vi "UHR-Fleezers Control (host) - 10.6.vi"() -> ()   [LabVIEW 2011] (continued)
        n1265 = Open/Create/Replace File(file path (use dialog)=w1906, operation (0:open)=T25."open", access (0:read/write)=enum16{"read/write", "read-only", "write-only"}."read-only") -> (refnum out=w1914:refnum<file>, error out=w1900:errorcluster)  [unwired: 1 in, 3 out]
        n1266 = Deny Access(4:w1900, 7:w1914) -> (0:w1899:errorcluster, 3:w1905:refnum<file>)  [unwired: 1 out]
        n1267 = Read from Binary File(5:0.0, 8:w1899, 9:T24."big-endian, network order" ("byte order (0:big-endian, network order)"), 10:-1 ("count (1)"), 11:w1905) -> (0:w1898:errorcluster, 2:w1896:dbl[], 3:w1901:refnum<file>)  [unwired: 2 out]
        n1268 = Array To Cluster(array=w1896) -> (cluster=w1895:T27)
        n1269 = Unbundle(w1895) -> ("[0]"=w1894:dbl, "[1]"=w1893:dbl, "[2]"=w1892:dbl, "[3]"=w1891:dbl, "[4]"=w1890:dbl, "[5]"=w1889:dbl)
        n1270 = Close File(refnum=w1901, error in=w1898) -> (error out=→"Read cal error":errorcluster)  [unwired: 1 out]
        n1271 = Multiply(x=w1889, y=w1886) -> (x*y=w1887:dbl)
        n1272 = local write "T2 kappa_x (pN/nm)"(w1891) -> ()
        n1273 = local write "T1 kappa_x (pN/nm)"(w1892) -> ()
        n1274 = local write "T1 alpha_x (nm/V)"(w1894) -> ()
        n1275 = local write "T2 alpha_x (nm/V)"(w1893) -> ()
        n1276 = Multiply(x=w1890, y=w1886) -> (x*y=w1888:dbl)
        n1277 = local write "T1 offset_x (mV)"(w1888) -> ()
        n1278 = local write "T2 offset_x (mV)"(w1887) -> ()
      }
      event "Abort MCL Scan": Value Change {
        n1279 = event-data() -> ()  [unwired: 7 out]
        n1280 = local write "MCL Scanning"(FALSE ("MCL Scanning")) -> ()
        n1281 = xnode "Read/Write Control"("FPGA VI Reference In"=w1919, "error in"=w1918, "Abort scan (MCL)"="Abort MCL Scan") -> ("error out"=w1917:errorcluster)  [unwired: 1 out]
      }
      event "Update Count (MCL)": Value Change {
        n1282 = event-data() -> ()  [unwired: 7 out]
        n1283 = xnode "Read/Write Control"("FPGA VI Reference In"=w1923, "error in"=w1922, "MCL count"="Update Count (MCL)") -> ("error out"=w1921:errorcluster)  [unwired: 1 out]
      }
      event "Phase adjust (MCL)", "+ phase (MCL)", "- phase (MCL)": Value Change {
        n1284 = event-data() -> ()  [unwired: 7 out]
        n1285 = Negate(x="Phase adjust (MCL)") -> (-x=w1932:i16)
        n1286 = Select(t=w1932, s="- phase (MCL)", f="Phase adjust (MCL)") -> (s? t:f=w1930:i16)
        n1287 = Or(x="- phase (MCL)", y="+ phase (MCL)") -> (x .or. y?=w1925:bool)
        n1288 = xnode "Read/Write Control"("FPGA VI Reference In"=w1934, "error in"=w1933, "Phase count adjustment (MCL)"=w1930) -> ("FPGA VI Reference Out"=w1926:T19, "error out"=w1927:errorcluster)
        n1289 = xnode "Read/Write Control"("FPGA VI Reference In"=w1926, "error in"=w1927, "+ phase (MCL)"=w1925) -> ("error out"=w1924:errorcluster)  [unwired: 1 out]
      }
      event "Abort AOD Scan": Value Change {
        n1290 = event-data() -> ()  [unwired: 7 out]
        n1291 = xnode "Read/Write Control"("FPGA VI Reference In"=w1938, "error in"=w1937, "Abort scan"="Abort AOD Scan") -> ("error out"=w1936:errorcluster)  [unwired: 1 out]
      }
      event "Continuous AOD Scanning": Value Change {
        n1292 = event-data() -> ()  [unwired: 7 out]
        n1293 = xnode "Read/Write Control"("FPGA VI Reference In"=w1942, "error in"=w1941, "Cont. Scan"="Continuous AOD Scanning") -> ("error out"=w1940:errorcluster)  [unwired: 1 out]
      }
      event "Index": Value Change {
        n1294 = event-data() -> ()  [unwired: 7 out]
        n1295 = call "Create new save file.vi"("Insert"="", "Ext"=".dat" ("string"), "Index In"="Index") -> ("Path Out"=→"Save file name":path, "Index Out"=w1943:dbl)
        "Save index" <- w1943
        n1296 = local write "Index"(w1943) -> ()
      }
      event "AO1", "AO2": Value Change {
        w1958 = 10.0 ("y")
        w1957 = 32767.0 ("y")
        n1297 = event-data() -> ()  [unwired: 7 out]
        n1298 = local read "AO2"() -> (w1956:dbl)
        n1299 = local read "AO1"() -> (w1953:dbl)
        n1300 = Multiply(x=w1953, y=w1957) -> (x*y=w1952:dbl)
        n1301 = Multiply(x=w1956, y=w1957) -> (x*y=w1955:dbl)
        n1302 = Divide(x=w1952, y=w1958) -> (x/y=w1951:dbl)
        n1303 = Divide(x=w1955, y=w1958) -> (x/y=w1954:dbl)
        n1304 = To Word Integer(number=w1951) -> (16bit integer=w1959:i16)
        n1305 = To Word Integer(number=w1954) -> (16bit integer=w1960:i16)
        n1306 = xnode "Read/Write Control"("FPGA VI Reference In"=w1950, "error in"=w1949, "AO1"=w1959, "AO2"=w1960) -> ("error out"=w1948:errorcluster)  [unwired: 1 out]
      }
      event "Inject Pump 1": Value Change {
        n1307 = event-data() -> ()  [unwired: 7 out]
        n1308 = local read "Use Harvard pumps\nfor beads (else Chemyx)"() -> (w1962:bool)
        n1309 = case shown="True" w1962 {
          tunnel: "Inject Pump 1" -> [w1966 w2004]
          tunnel: w1961 -> [_ w2005]
          frame False {
            n1310 = local read "Pump write delay (ms)"() -> (w1965:dbl)
            n1311 = local read "Chemyx Syringe Pump Serial Port"() -> (w1964:refnum<visa-resource-name>)
            n1312 = case shown="True" w1966 {
              tunnel: w1965 -> [w1972 w1986]
              tunnel: w1964 -> [w1969 w1985]
              frame False {
                n1313 = flat-sequence {
                  tunnel: w1969 -> [w1973]
                  tunnel: [w1973] -> w1970
                  tunnel: w1972 -> [_]
                  tunnel: [w1976] -> w1971
                  tunnel: w1970 -> [w1976]
                  tunnel: w1971 -> [w1977]
                  tunnel: [w1977] -> w1967
                  tunnel: [w1979] -> w1968
                  tunnel: w1967 -> [w1979]
                  tunnel: w1968 -> [w1981]
                  frame #0 {
                    n1314 = call "Write to pump.vi"("string"="enter pump1", "VISA resource name"=w1973) -> ()  [unwired: 1 out]
                  }
                  frame #1 {
                    n1315 = Wait (ms)(milliseconds to wait="Pump pause delay (ms)") -> ()  [unwired: 1 out]
                  }
                  frame #2 {
                    n1316 = call "Write to pump.vi"("string"="stop", "VISA resource name"=w1977) -> ()  [unwired: 1 out]
                  }
                  frame #3 {
                    n1317 = Wait (ms)(milliseconds to wait=u32 500) -> ()  [unwired: 1 out]
                  }
                  frame #4 {
                    n1318 = call "Write to pump.vi"("string"="stop", "VISA resource name"=w1981) -> ()  [unwired: 1 out]
                  }
                }
              }
              frame True {
                n1319 = flat-sequence {
                  tunnel: w1985 -> [w1995]
                  tunnel: w1986 -> [w1990]
                  tunnel: w1986 -> [w1997]
                  tunnel: w1985 -> [w1998]
                  tunnel: [w1998] -> w1983
                  tunnel: [w2000] -> w1984
                  tunnel: w1983 -> [w2000]
                  tunnel: w1984 -> [w2002]
                  frame #0 {
                    n1320 = local read "All Pump Parameters"() -> (w1989:T5)
                    n1321 = Unbundle By Name(w1989) -> ("Pump 1"=w1996:T28)
                    n1322 = call "Set pump parameters.vi"("Pump write delay (ms)"=w1990, "Volume (uL)"="Ch 1 Inject Volume (uL)", "Rate (uL/h)"="Ch 1 Inject Rate (ul/h)", "Units"=4.0, "Pump #"=1.0, "Pump Parameters In"=w1996, "VISA resource name"=w1995) -> ("Pump Parameters Out"=w1988:T28)  [unwired: 3 in]
                    n1323 = Bundle By Name(cluster=w1989, "Pump 1"=w1988) -> (w1987:T5)
                    n1324 = local write "All Pump Parameters"(w1987) -> ()
                  }
                  frame #1 {
                    n1325 = Wait (ms)(milliseconds to wait=w1997) -> ()  [unwired: 1 out]
                  }
                  frame #2 {
                    n1326 = call "Write to pump.vi"("string"="start", "VISA resource name"=w1998) -> ()  [unwired: 1 out]
                  }
                  frame #3 {
                    n1327 = Wait (ms)(milliseconds to wait=u32 500) -> ()  [unwired: 1 out]
                  }
                  frame #4 {
                    n1328 = call "Write to pump.vi"("string"="start", "VISA resource name"=w2002) -> ()  [unwired: 1 out]
                  }
                }
              }
            }
          }
          frame True {
            n1329 = case shown="False" w2004 {
              tunnel: w2005 -> [w2006 w2016]
              frame False {
                n1330 = flat-sequence {
                  tunnel: w2006 -> [w2008]
                  frame #0 {
                    n1331 = local write "Flushing P1"(FALSE ("Flushing P1")) -> ()
                    n1332 = Concatenate Strings("stop" ("string"), "\r") -> (w2010:string)
                    n1333 = VISA Write(VISA resource name=w2008, write buffer=w2010) -> ()  [unwired: 1 in, 3 out]
                  }
                  frame #1 {
                    n1334 = property on="Clear Volume P1" class="Bool (strict)"("Val(Sgnl)"=TRUE ("Value (Signaling)")) -> ()  [unwired: 2 in, 2 out]
                  }
                }
              }
              frame True {
                n1335 = local read "Normal Flow Rate (ul/h) P1"() -> (w2014:dbl)
                n1336 = Number To Decimal String(number=w2014) -> (decimal integer string=w2020:string)  [unwired: 1 in]
                n1337 = Concatenate Strings("irate  " ("string"), w2020, " u/h" ("string"), "\r") -> (w2018:string)
                n1338 = VISA Write(VISA resource name=w2016, write buffer=w2018) -> (VISA resource name out=w2015:refnum<visa-resource-name>)  [unwired: 1 in, 2 out]
                n1339 = Concatenate Strings("irun" ("string"), "\r") -> (w2022:string)
                n1340 = VISA Write(VISA resource name=w2015, write buffer=w2022) -> ()  [unwired: 1 in, 3 out]
              }
            }
          }
        }
      }
      event "Inject Pump 3": Value Change {
        n1341 = event-data() -> ()  [unwired: 7 out]
        n1342 = local read "Use Harvard pumps\nfor beads (else Chemyx)"() -> (w2025:bool)
        n1343 = case shown="True" w2025 {
          tunnel: "Inject Pump 3" -> [w2029 w2068]
          tunnel: w2024 -> [_ w2067]
          frame False {
            n1344 = local read "Pump write delay (ms)"() -> (w2028:dbl)
            n1345 = case shown="True" w2029 {
              tunnel: w2028 -> [w2035 w2049]
              tunnel: "Chemyx Syringe Pump Serial Port" -> [w2032 w2048]
              frame False {
                n1346 = flat-sequence {
                  tunnel: w2032 -> [w2036]
                  tunnel: [w2036] -> w2033
                  tunnel: w2035 -> [_]
                  tunnel: [w2039] -> w2034
                  tunnel: w2033 -> [w2039]
                  tunnel: w2034 -> [w2040]
                  tunnel: [w2040] -> w2030
                  tunnel: [w2042] -> w2031
                  tunnel: w2030 -> [w2042]
                  tunnel: w2031 -> [w2044]
                  frame #0 {
                    n1347 = call "Write to pump.vi"("string"="enter pump3", "VISA resource name"=w2036) -> ()  [unwired: 1 out]
                  }
                  frame #1 {
                    n1348 = local read "Pump pause delay (ms)"() -> (w2038:u32)
                    n1349 = Wait (ms)(milliseconds to wait=w2038) -> ()  [unwired: 1 out]
                  }
                  frame #2 {
                    n1350 = call "Write to pump.vi"("string"="stop", "VISA resource name"=w2040) -> ()  [unwired: 1 out]
                  }
                  frame #3 {
                    n1351 = Wait (ms)(milliseconds to wait=u32 0) -> ()  [unwired: 1 out]
                  }
                  frame #4 {
                    n1352 = call "Write to pump.vi"("string"="stop", "VISA resource name"=w2044) -> ()  [unwired: 1 out]
                  }
                }
              }
              frame True {
                n1353 = flat-sequence {
                  tunnel: w2048 -> [w2058]
                  tunnel: w2049 -> [w2053]
                  tunnel: w2049 -> [w2060]
                  tunnel: w2048 -> [w2061]
                  tunnel: [w2061] -> w2047
                  tunnel: [w2064] -> w2046
                  tunnel: w2047 -> [w2064]
                  tunnel: w2046 -> [w2065]
                  frame #0 {
                    n1354 = local read "All Pump Parameters"() -> (w2052:T5)
                    n1355 = Unbundle By Name(w2052) -> ("Pump 3"=w2059:T28)
                    n1356 = call "Set pump parameters.vi"("Pump write delay (ms)"=w2053, "Volume (uL)"="Ch 3 Inject Volume (uL)", "Rate (uL/h)"="Ch 3 Inject Rate (ul/h)", "Units"=4.0, "Pump #"=3.0, "Pump Parameters In"=w2059, "VISA resource name"=w2058) -> ("Pump Parameters Out"=w2051:T28)  [unwired: 3 in]
                    n1357 = Bundle By Name(cluster=w2052, "Pump 3"=w2051) -> (w2050:T5)
                    n1358 = local write "All Pump Parameters"(w2050) -> ()
                  }
                  frame #1 {
                    n1359 = Wait (ms)(milliseconds to wait=w2060) -> ()  [unwired: 1 out]
                  }
                  frame #2 {
                    n1360 = call "Write to pump.vi"("string"="start", "VISA resource name"=w2061) -> ()  [unwired: 1 out]
                  }
                  frame #3 {
                    n1361 = Wait (ms)(milliseconds to wait=u32 500) -> ()  [unwired: 1 out]
                  }
                  frame #4 {
                    n1362 = call "Write to pump.vi"("string"="start", "VISA resource name"=w2065) -> ()  [unwired: 1 out]
                  }
                }
              }
            }
          }
          frame True {
            n1363 = case shown="False" w2068 {
              tunnel: w2067 -> [w2069 w2076]
              frame False {
                n1364 = flat-sequence {
                  tunnel: w2069 -> [w2071]
                  frame #0 {
                    n1365 = local write "Flushing P3"(FALSE ("Flushing P3")) -> ()
                    n1366 = Concatenate Strings("stop" ("string"), "\r") -> (w2073:string)
                    n1367 = VISA Write(VISA resource name=w2071, write buffer=w2073) -> ()  [unwired: 1 in, 3 out]
                  }
                  frame #1 {
                    n1368 = property on="Clear Volume P3" class="Bool (strict)"("Val(Sgnl)"=TRUE ("Value (Signaling)")) -> ()  [unwired: 2 in, 2 out]
                  }
                }
              }
              frame True {
                n1369 = local read "Normal Flow Rate (ul/h) P3"() -> (w2077:dbl)
                n1370 = Number To Decimal String(number=w2077) -> (decimal integer string=w2083:string)  [unwired: 1 in]
                n1371 = Concatenate Strings("irate  " ("string"), w2083, " u/h" ("string"), "\r") -> (w2081:string)
                n1372 = VISA Write(VISA resource name=w2076, write buffer=w2081) -> (VISA resource name out=w2079:refnum<visa-resource-name>)  [unwired: 1 in, 2 out]
                n1373 = Concatenate Strings("irun" ("string"), "\r") -> (w2085:string)
                n1374 = VISA Write(VISA resource name=w2079, write buffer=w2085) -> ()  [unwired: 1 in, 3 out]
              }
            }
          }
        }
      }
      event "Inject Pump 2": Value Change {
        n1375 = event-data() -> ()  [unwired: 7 out]
        n1376 = local read "Pump write delay (ms)"() -> (w2089:dbl)
        n1377 = flat-sequence {
          tunnel: w2087 -> [w2102]
          tunnel: w2089 -> [w2098]
          tunnel: "Inject Pump 2" -> [_]
          tunnel: w2089 -> [w2104]
          tunnel: w2087 -> [w2105]
          frame #0 {
            n1378 = local read "All Pump Parameters"() -> (w2097:T5)
            n1379 = Multiply(x=60.0, y="Flush Center Ch Rate (ul/m)") -> (x*y=w2094:dbl)
            n1380 = Unbundle By Name(w2097) -> ("Pump 2"=w2103:T28)
            n1381 = call "Set pump parameters.vi"("Pump write delay (ms)"=w2098, "Volume (uL)"="Flush Center Ch Volume (uL)", "Rate (uL/h)"=w2094, "Units"=3.0, "Pump #"=2.0, "Pump Parameters In"=w2103, "VISA resource name"=w2102) -> ("Pump Parameters Out"=w2096:T28)  [unwired: 3 in]
            n1382 = Bundle By Name(cluster=w2097, "Pump 2"=w2096) -> (w2095:T5)
            n1383 = local write "All Pump Parameters"(w2095) -> ()
            n1384 = Add(x="Flush Center Ch Volume (uL)", y="Total Volume\nFlushed (uL)") -> (x+y=w2091:dbl)
            n1385 = local write "Total Volume\nFlushed (uL)"(w2091) -> ()
          }
          frame #1 {
            n1386 = Wait (ms)(milliseconds to wait=w2104) -> ()  [unwired: 1 out]
          }
          frame #2 {
            n1387 = call "Write to pump.vi"("string"="start", "VISA resource name"=w2105) -> ()  [unwired: 1 out]
          }
        }
        n1388 = local read "Chemyx Syringe Pump Serial Port"() -> (w2087:refnum<visa-resource-name>)
      }
      event "Sample Channel\nFlow": Value Change {
        n1389 = event-data() -> ()  [unwired: 7 out]
        n1390 = Select(t="irun" ("string"), s="Sample Channel\nFlow", f="stop" ("string")) -> (s? t:f=w2109:string)
        n1391 = Concatenate Strings(w2109, "\r") -> (w2112:string)
        n1392 = VISA Write(VISA resource name=w2107, write buffer=w2112) -> ()  [unwired: 1 in, 3 out]
      }
      event "Start Flow": Value Change {
        n1393 = event-data() -> ()  [unwired: 7 out]
        n1394 = local write "Sample Channel\nFlow"(TRUE ("Sample Channel\nFlow")) -> ()
        n1395 = local write "Start Flow"(FALSE ("Start Flow")) -> ()
        n1396 = Concatenate Strings("irun" ("string"), "\r") -> (w2118:string)
        n1397 = VISA Write(VISA resource name=w2114, write buffer=w2118) -> ()  [unwired: 1 in, 3 out]
      }
      event "Stop Flow": Value Change {
        w2120 = FALSE ("Stop Flow")
        n1398 = event-data() -> ()  [unwired: 7 out]
        n1399 = local write "Stop Flow"(w2120) -> ()
        n1400 = local write "Sample Channel\nFlow"(w2120) -> ()
        n1401 = Concatenate Strings("stop" ("string"), "\r") -> (w2123:string)
        n1402 = VISA Write(VISA resource name=w2121, write buffer=w2123) -> ()  [unwired: 1 in, 3 out]
      }
      event "Flow rate (uL/h)": Value Change {
        n1403 = event-data() -> ()  [unwired: 7 out]
        n1404 = Number To Decimal String(number="Flow rate (uL/h)") -> (decimal integer string=w2130:string)  [unwired: 1 in]
        n1405 = Concatenate Strings("irate  " ("string"), w2130, " u/h" ("string"), "\r") -> (w2129:string)
        n1406 = VISA Write(VISA resource name=w2126, write buffer=w2129) -> ()  [unwired: 1 in, 3 out]
      }
      event "Flush Sample": Value Change {
        n1407 = event-data() -> ()  [unwired: 7 out]
        n1408 = flat-sequence {
          tunnel: w2135 -> [w2163]
          tunnel: [w2143] -> w2134
          tunnel: [w2137] -> w2132
          tunnel: w2134 -> [w2167]
          tunnel: [w2167] -> w2133
          tunnel: w2132 -> [w2166]
          tunnel: w2133 -> [w2172]
          frame #0 {
            # "set paramaters (rate, volume) for flush, clear volume"
            n1409 = Number To Decimal String(number="Flush rate (uL/m)") -> (decimal integer string=w2159:string)  [unwired: 1 in]
            n1410 = Concatenate Strings("irate  " ("string"), w2159, " u/m" ("string"), "\r") -> (w2161:string)
            n1411 = VISA Write(VISA resource name=w2163, write buffer=w2161) -> (VISA resource name out=w2157:refnum<visa-resource-name>)  [unwired: 1 in, 2 out]
            n1412 = Reciprocal(x="Flush rate (uL/m)") -> (1/x=w2140:dbl)
            n1413 = Number To Decimal String(number="Volume (uL)") -> (decimal integer string=w2148:string)  [unwired: 1 in]
            n1414 = Multiply(x="Volume (uL)", y=w2140) -> (x*y=w2139:dbl)
            n1415 = Concatenate Strings("tvolume  " ("string"), w2148, " u" ("string"), "\r") -> (w2146:string)
            n1416 = Multiply(x=w2139, y=60000.0) -> (x*y=w2137:dbl)
            n1417 = VISA Write(VISA resource name=w2157, write buffer=w2146) -> (VISA resource name out=w2145:refnum<visa-resource-name>)  [unwired: 1 in, 2 out]
            n1418 = Concatenate Strings("cvolume" ("string"), "\r") -> (w2144:string)
            n1419 = VISA Write(VISA resource name=w2145, write buffer=w2144) -> (VISA resource name out=w2155:refnum<visa-resource-name>)  [unwired: 1 in, 2 out]
            n1420 = Concatenate Strings("irun" ("string"), "\r") -> (w2153:string)
            n1421 = VISA Write(VISA resource name=w2155, write buffer=w2153) -> (VISA resource name out=w2143:refnum<visa-resource-name>)  [unwired: 1 in, 2 out]
          }
          frame #1 {
            # "Have to wait until\nflow is done to reset\nrate"
            n1422 = Add(x=w2166, y=100.0) -> (x+y=w2165:dbl)
            n1423 = Wait (ms)(milliseconds to wait=w2165) -> ()  [unwired: 1 out]
          }
          frame #2 {
            # "reset flow rate to usual flow rate"
            n1424 = local read "Flow rate (uL/h)"() -> (w2178:dbl)
            n1425 = Number To Decimal String(number=w2178) -> (decimal integer string=w2176:string)  [unwired: 1 in]
            n1426 = Concatenate Strings("irate  " ("string"), w2176, " u/h" ("string"), "\r") -> (w2174:string)
            n1427 = VISA Write(VISA resource name=w2172, write buffer=w2174) -> (VISA resource name out=w2168:refnum<visa-resource-name>)  [unwired: 1 in, 2 out]
            n1428 = Concatenate Strings("cvolume" ("string"), "\r") -> (w2169:string)
            n1429 = VISA Write(VISA resource name=w2168, write buffer=w2169) -> ()  [unwired: 1 in, 3 out]
          }
        }
      }
      event "Flush Pump 3": Value Change {
        n1430 = event-data() -> ()  [unwired: 7 out]
        n1431 = flat-sequence {
          tunnel: w2179 -> [w2182]
          frame #0 {
            # "set paramaters (rate, volume) for flush, clear volume"
            n1432 = Number To Decimal String(number="Flush rate (uL/m) P3") -> (decimal integer string=w2204:string)  [unwired: 1 in]
            n1433 = local write "Inject Pump 3"(TRUE ("Inject Pump 3")) -> ()
            n1434 = Concatenate Strings("irate  " ("string"), w2204, " u/m" ("string"), "\r") -> (w2206:string)
            n1435 = VISA Write(VISA resource name=w2182, write buffer=w2206) -> (VISA resource name out=w2202:refnum<visa-resource-name>)  [unwired: 1 in, 2 out]
            n1436 = Reciprocal(x="Flush rate (uL/m) P3") -> (1/x=w2186:dbl)
            n1437 = Number To Decimal String(number="Volume (uL) P3") -> (decimal integer string=w2193:string)  [unwired: 1 in]
            n1438 = Multiply(x="Volume (uL) P3", y=w2186) -> (x*y=w2185:dbl)
            n1439 = Concatenate Strings("tvolume  " ("string"), w2193, " u" ("string"), "\r") -> (w2191:string)
            n1440 = Multiply(x=w2185, y=60.0) -> (x*y=→"HP3 Flush Time (s)":dbl)
            n1441 = VISA Write(VISA resource name=w2202, write buffer=w2191) -> (VISA resource name out=w2190:refnum<visa-resource-name>)  [unwired: 1 in, 2 out]
            n1442 = Concatenate Strings("cvolume" ("string"), "\r") -> (w2189:string)
            n1443 = VISA Write(VISA resource name=w2190, write buffer=w2189) -> (VISA resource name out=w2200:refnum<visa-resource-name>)  [unwired: 1 in, 2 out]
            n1444 = Concatenate Strings("irun" ("string"), "\r") -> (w2198:string)
            n1445 = VISA Write(VISA resource name=w2200, write buffer=w2198) -> ()  [unwired: 1 in, 3 out]
          }
          frame #1 {
            "Flushing P3" <- TRUE ("Flushing P3")
          }
        }
      }
      event "Flush Pump 1": Value Change {
        n1446 = event-data() -> ()  [unwired: 7 out]
        n1447 = flat-sequence {
          tunnel: [w2220] -> w2210
          tunnel: w2209 -> [w2213]
          tunnel: w2210 -> [_]
          frame #0 {
            # "set paramaters (rate, volume) for flush, clear volume"
            n1448 = local write "Inject Pump 1"(TRUE ("Inject Pump 1")) -> ()
            n1449 = Number To Decimal String(number="Flush rate (uL/m) P1") -> (decimal integer string=w2236:string)  [unwired: 1 in]
            n1450 = Concatenate Strings("irate  " ("string"), w2236, " u/m" ("string"), "\r") -> (w2238:string)
            n1451 = VISA Write(VISA resource name=w2213, write buffer=w2238) -> (VISA resource name out=w2234:refnum<visa-resource-name>)  [unwired: 1 in, 2 out]
            n1452 = Reciprocal(x="Flush rate (uL/m) P1") -> (1/x=w2217:dbl)
            n1453 = Number To Decimal String(number="Volume (uL) P1") -> (decimal integer string=w2225:string)  [unwired: 1 in]
            n1454 = Multiply(x="Volume (uL) P1", y=w2217) -> (x*y=w2216:dbl)
            n1455 = Concatenate Strings("tvolume  " ("string"), w2225, " u" ("string"), "\r") -> (w2223:string)
            n1456 = Multiply(x=w2216, y=60.0) -> (x*y=→"HP1 Flush Time (s)":dbl)
            n1457 = VISA Write(VISA resource name=w2234, write buffer=w2223) -> (VISA resource name out=w2222:refnum<visa-resource-name>)  [unwired: 1 in, 2 out]
            n1458 = Concatenate Strings("cvolume" ("string"), "\r") -> (w2221:string)
            n1459 = VISA Write(VISA resource name=w2222, write buffer=w2221) -> (VISA resource name out=w2232:refnum<visa-resource-name>)  [unwired: 1 in, 2 out]
            n1460 = Concatenate Strings("irun" ("string"), "\r") -> (w2230:string)
            n1461 = VISA Write(VISA resource name=w2232, write buffer=w2230) -> (VISA resource name out=w2220:refnum<visa-resource-name>)  [unwired: 1 in, 2 out]
          }
          frame #1 {
            "Flushing P1" <- TRUE ("Flushing P3")
          }
        }
      }
      event "Clear Volume": Value Change {
        n1462 = event-data() -> ()  [unwired: 7 out]
        n1463 = Concatenate Strings("cvolume" ("string"), "\r") -> (w2242:string)
        n1464 = VISA Write(VISA resource name=w2241, write buffer=w2242) -> ()  [unwired: 1 in, 3 out]
      }
      event "Clear Volume P3": Value Change {
        n1465 = event-data() -> ()  [unwired: 7 out]
        n1466 = Concatenate Strings("cvolume" ("string"), "\r") -> (w2248:string)
        n1467 = VISA Write(VISA resource name=w2247, write buffer=w2248) -> ()  [unwired: 1 in, 3 out]
        n1468 = local write "Clear Volume P3"(FALSE ("Clear Volume P3")) -> ()
      }
      event "Clear Volume P1": Value Change {
        n1469 = event-data() -> ()  [unwired: 7 out]
        n1470 = Concatenate Strings("cvolume" ("string"), "\r") -> (w2253:string)
        n1471 = local write "Clear Volume P1"(FALSE ("Clear Volume P1")) -> ()
        n1472 = VISA Write(VISA resource name=w2252, write buffer=w2253) -> ()  [unwired: 1 in, 3 out]
      }
      event "Display On P3": Value Change {
        n1473 = event-data() -> ()  [unwired: 7 out]
        n1474 = Select(t="dim 100", s="Display On P3", f="dim 0") -> (s? t:f=w2259:string)
        n1475 = Concatenate Strings(w2259, "\r") -> (w2261:string)
        n1476 = VISA Write(VISA resource name=w2256, write buffer=w2261) -> ()  [unwired: 1 in, 3 out]
      }
      event "Display On P1": Value Change {
        n1477 = event-data() -> ()  [unwired: 7 out]
        n1478 = Select(t="dim 100", s="Display On P1", f="dim 0") -> (s? t:f=w2266:string)
        n1479 = Concatenate Strings(w2266, "\r") -> (w2268:string)
        n1480 = VISA Write(VISA resource name=w2263, write buffer=w2268) -> ()  [unwired: 1 in, 3 out]
      }
      event "Retract Pump 3": Value Change {
        n1481 = event-data() -> ()  [unwired: 7 out]
        n1482 = local write "Retract Pump 3"(FALSE ("Retract Pump 3")) -> ()
        n1483 = case shown="True" "Retract Pump 3" {
          tunnel: w2270 -> [_ w2273]
          frame False {
          }
          frame True {
            n1484 = Number To Decimal String(number="Retract Rate (uL/m)") -> (decimal integer string=w2291:string)  [unwired: 1 in]
            n1485 = Concatenate Strings("wrate  " ("string"), w2291, " u/m" ("string"), "\r") -> (w2293:string)
            n1486 = VISA Write(VISA resource name=w2273, write buffer=w2293) -> (VISA resource name out=w2284:refnum<visa-resource-name>)  [unwired: 1 in, 2 out]
            n1487 = Number To Decimal String(number="Retract Vol 3 (uL)") -> (decimal integer string=w2286:string)  [unwired: 1 in]
            n1488 = Concatenate Strings("tvolume  " ("string"), w2286, " u" ("string"), "\r") -> (w2283:string)
            n1489 = VISA Write(VISA resource name=w2284, write buffer=w2283) -> (VISA resource name out=w2279:refnum<visa-resource-name>)  [unwired: 1 in, 2 out]
            n1490 = Concatenate Strings("cvolume" ("string"), "\r") -> (w2280:string)
            n1491 = VISA Write(VISA resource name=w2279, write buffer=w2280) -> (VISA resource name out=w2274:refnum<visa-resource-name>)  [unwired: 1 in, 2 out]
            n1492 = Concatenate Strings("wrun" ("string"), "\r") -> (w2275:string)
            n1493 = VISA Write(VISA resource name=w2274, write buffer=w2275) -> ()  [unwired: 1 in, 3 out]
          }
        }
      }
      event "Retract Pump 1": Value Change {
        n1494 = event-data() -> ()  [unwired: 7 out]
        n1495 = local write "Retract Pump 1"(FALSE ("Retract Pump 1")) -> ()
        n1496 = case shown="True" "Retract Pump 1" {
          tunnel: w2295 -> [_ w2300]
          frame False {
          }
          frame True {
            n1497 = local read "Retract Rate (uL/m)"() -> (w2298:dbl)
            n1498 = Number To Decimal String(number=w2298) -> (decimal integer string=w2316:string)  [unwired: 1 in]
            n1499 = Concatenate Strings("wrate  " ("string"), w2316, " u/m" ("string"), "\r") -> (w2318:string)
            n1500 = VISA Write(VISA resource name=w2300, write buffer=w2318) -> (VISA resource name out=w2310:refnum<visa-resource-name>)  [unwired: 1 in, 2 out]
            n1501 = Number To Decimal String(number="Retract Vol 1 (uL)") -> (decimal integer string=w2312:string)  [unwired: 1 in]
            n1502 = Concatenate Strings("tvolume  " ("string"), w2312, " u" ("string"), "\r") -> (w2309:string)
            n1503 = VISA Write(VISA resource name=w2310, write buffer=w2309) -> (VISA resource name out=w2306:refnum<visa-resource-name>)  [unwired: 1 in, 2 out]
            n1504 = Concatenate Strings("cvolume" ("string"), "\r") -> (w2307:string)
            n1505 = VISA Write(VISA resource name=w2306, write buffer=w2307) -> (VISA resource name out=w2301:refnum<visa-resource-name>)  [unwired: 1 in, 2 out]
            n1506 = Concatenate Strings("wrun" ("string"), "\r") -> (w2302:string)
            n1507 = VISA Write(VISA resource name=w2301, write buffer=w2302) -> ()  [unwired: 1 in, 3 out]
          }
        }
      }
      event "Flip Green Filter": Value Change {
        n1508 = event-data() -> ()  [unwired: 7 out]
        n1509 = Not(x="Flip Green Filter") -> (.not. x?=w2320:bool)
        n1510 = local write "Flip Green Filter"(w2320) -> ()
        n1511 = flat-sequence {
          tunnel: w2328 -> [w2333]
          tunnel: w2327 -> [w2332]
          tunnel: [w2330] -> w2325
          tunnel: [w2329] -> w2324
          tunnel: [w2335] -> w2323
          tunnel: w2325 -> [w2335]
          tunnel: [w2334] -> w2322
          tunnel: w2324 -> [w2334]
          tunnel: w2323 -> [w2339]
          tunnel: w2322 -> [w2338]
          tunnel: [w2337] -> w2326
          frame #0 {
            n1512 = xnode "Read/Write Control"("FPGA VI Reference In"=w2333, "error in"=w2332, "Green Filter Flipper"=TRUE) -> ("FPGA VI Reference Out"=w2330:T19, "error out"=w2329:errorcluster)
          }
          frame #1 {
            n1513 = Wait (ms)(milliseconds to wait=u32 100) -> ()  [unwired: 1 out]
          }
          frame #2 {
            n1514 = xnode "Read/Write Control"("FPGA VI Reference In"=w2339, "error in"=w2338, "Green Filter Flipper"=FALSE) -> ("error out"=w2337:errorcluster)  [unwired: 1 out]
          }
        }
      }
      event "Pump 1 contents", "Pump 3 contents": Value Change {
        n1515 = event-data() -> ()  [unwired: 7 out]
        n1516 = local read "Pump 1 contents"() -> (→"Pump 1 cont disp":string)
        n1517 = local read "Pump 3 contents"() -> (→"Pump 3 cont disp":string)
      }
      event "Reset Trap Pos. FB": Value Change {
        n1518 = event-data() -> ()  [unwired: 7 out]
        n1519 = xnode "Read/Write Control"("FPGA VI Reference In"=w2345, "error in"=w2344, "Trap Pos. FB Reset"="Reset Trap Pos. FB") -> ()  [unwired: 2 out]
      }
      event "Rem fb disp offset": Value Change {
        n1520 = event-data() -> ()  [unwired: 7 out]
        n1521 = local write "Rem fb disp offset"(FALSE ("Rem fb disp offset")) -> ()
        n1522 = local read "Mean T1 Position (nm)"() -> (w2347:dbl)
        n1523 = local read "FB Trap Pos Offset"() -> (w2348:dbl)
        n1524 = Subtract(x=w2348, y=w2347) -> (x-y=w2346:dbl)
        n1525 = local write "FB Trap Pos Offset"(w2346) -> ()
      }
      event "Threshold (nm)": Value Change {
        n1526 = event-data() -> ()  [unwired: 7 out]
        n1527 = flat-sequence {
          tunnel: w2352 -> [w2360]
          tunnel: w2351 -> [w2359]
          tunnel: [w2353] -> w2350
          tunnel: w2350 -> [w2366]
          frame #0 {
            n1528 = xnode "Read/Write Control"("FPGA VI Reference In"=w2360, "error in"=w2359) -> ("FPGA VI Reference Out"=w2356:T19, "error out"=w2355:errorcluster, "FPGA TTrig Thresh"=w2357:i64)
            n1529 = local read "Threshold stored (nm)"() -> (w2365:dbl)
            n1530 = local read "Threshold (nm)"() -> (w2353:dbl)
            n1531 = local read "AOM X Cal (nm/MHz)"() -> (w2363:dbl)
            n1532 = Subtract(x=w2353, y=w2365) -> (x-y=w2364:dbl)
            n1533 = Divide(x=w2364, y=w2363) -> (x/y=w2361:dbl)
            n1534 = call "IR AOM freq to word.vi"("Frequency In (MHz)"=w2361) -> ("Frequency Word Out (double)"=w2362:dbl)
            n1535 = To Quad Integer(1:w2362) -> (0:w2358:i64)
            n1536 = Add(x=w2357, y=w2358) -> (x+y=w2354:i64)
            n1537 = xnode "Read/Write Control"("FPGA VI Reference In"=w2356, "error in"=w2355, "FPGA TTrig Thresh"=w2354) -> ()  [unwired: 2 out]
          }
          frame #1 {
            "Threshold stored (nm)" <- w2366
          }
        }
      }
      event "FB Trig Integrate": Value Change {
        n1538 = event-data() -> ()  [unwired: 7 out]
        n1539 = local read "FB Trig Integrate"() -> (w2368:u32)
        n1540 = xnode "Read/Write Control"("FPGA VI Reference In"=w2370, "error in"=w2369, "FB Trig Integrate"=w2368) -> ("error out"=w2367:errorcluster)  [unwired: 1 out]
      }
      event "11": Value Change {
        n1541 = event-data() -> ()  [unwired: 7 out]
        n1542 = local read "11"() -> (w2371:bool)
        n1543 = case shown="True" w2371 {
          frame False {
          }
          frame True {
            n1544 = local read "Messages"() -> (w2373:string)
            n1545 = call "Update messages.vi"("Message to add"="You kicked it up to 11!", "Old message string"=w2373) -> ("New message string"=w2374:string)
            n1546 = call <vilib>:"Beep.vi"() -> ()  [unwired: 12 in]
            n1547 = local write "Messages"(w2374) -> ()
          }
        }
      }
      event "Trap Pos. FB ON": Value Change {
        n1548 = event-data() -> ()  [unwired: 7 out]
        n1549 = xnode "Read/Write Control"("FPGA VI Reference In"=w2377, "error in"=w2376, "Force feedback"="Trap Pos. FB ON") -> ()  [unwired: 2 out]
      }
      event "Remove Action Offset": Value Change {
        n1550 = event-data() -> ()  [unwired: 7 out]
        n1551 = local write "Remove Action Offset"(FALSE ("Remove Action Offset")) -> ()
        n1552 = local read "Trap Pos. FB Mult Factor"() -> (w2382:i64)
        n1553 = local read "Trap Pos FB Action"() -> (w2380:i64)
        n1554 = local read "Trap Pos. FB Offset Factor"() -> (w2378:i64)
        n1555 = Multiply(x=w2382, y=w2380) -> (x*y=w2381:i64)
        n1556 = Add(x=w2381, y=w2378) -> (x+y=w2379:i64)
        n1557 = local write "Trap Pos. FB Offset Factor"(w2379) -> ()
        n1558 = xnode "Read/Write Control"("FPGA VI Reference In"=w2385, "error in"=w2384, "Trap Pos. FB Offset Factor"=w2379) -> ()  [unwired: 2 out]
      }
      event "Remove Unwinding Offset": Value Change {
        n1559 = event-data() -> ()  [unwired: 7 out]
        n1560 = local write "Remove Unwinding Offset"(FALSE ("Remove Action Offset")) -> ()
        n1561 = local read "Trap Pos. FB Mult Factor"() -> (w2397:i64)
        n1562 = local read "Trap Pos FB Action"() -> (w2395:i64)
        n1563 = local read "Trap Pos. FB Offset Factor"() -> (w2394:i64)
        n1564 = Multiply(x=w2397, y=w2395) -> (x*y=w2396:i64)
        n1565 = local read "Trap Pos. FB Mult Factor"() -> (w2393:i64)
        n1566 = Add(x=w2396, y=w2394) -> (x+y=w2387:i64)
        n1567 = Multiply(x=32768, y="factor") -> (x*y=w2390:dbl)
        n1568 = Multiply(x=w2390, y=w2393) -> (x*y=w2392:dbl)
        n1569 = Subtract(x=w2387, y=w2392) -> (x-y=w2391:dbl)
        n1570 = To Quad Integer(1:w2391) -> (0:w2386:i64)
        n1571 = xnode "Read/Write Control"("FPGA VI Reference In"=w2400, "error in"=w2399, "Trap Pos. FB Offset Factor"=w2386) -> ()  [unwired: 2 out]
        n1572 = local write "Trap Pos. FB Offset Factor"(w2386) -> ()
      }
      event "Trap Pos. FB Range", "Trap Pos. FB Gains", "Trap Pos. FB Mult Factor", "Trap Pos. FB Offset Factor", "Trap Pos FB Negate Action", "Trap Pos FB Monitor\nT1 or T2", "Differential FB?", "Negate Diff?": Value Change {
        n1573 = event-data() -> ()  [unwired: 7 out]
        n1574 = local read "Negate Diff?"() -> (w2401:bool)
        n1575 = xnode "Read/Write Control"("FPGA VI Reference In"=w2411, "error in"=w2410, "Trap Pos. FB Range"="Trap Pos. FB Range", "Trap Pos. FB Gains"="Trap Pos. FB Gains", "Trap Pos. FB Mult Factor"="Trap Pos. FB Mult Factor", "Trap Pos. FB Offset Factor"="Trap Pos. FB Offset Factor", "Trap Pos FB Negate Action"="Trap Pos FB Negate Action", "Trap Pos FB Monitor T1 or T2"="Trap Pos FB Monitor\nT1 or T2", "AI1 X Scale"="Trap Pos. AI1 X Pre-scale", "Negate Diff?"=w2401, "Diff FB Measurement?"="Differential FB?") -> ()  [unwired: 2 out]
      }
      event "Trap Pos FB SP": Value Change {
        n1576 = event-data() -> ()  [unwired: 7 out]
        n1577 = xnode "Read/Write Control"("FPGA VI Reference In"=w2414, "error in"=w2413, "Trap Pos. FB SP"="Trap Pos FB SP") -> ()  [unwired: 2 out]
      }
      event "Set Reading to\nSetpoint": Value Change {
        # "This is the actual PID input signal"
        n1578 = event-data() -> ()  [unwired: 7 out]
        n1579 = local write "Set Reading to\nSetpoint"(FALSE ("Set SP to Reading")) -> ()
        n1580 = xnode "Read/Write Control"("FPGA VI Reference In"=w2419, "error in"=w2418) -> ("FPGA VI Reference Out"=w2417:T19, "error out"=w2416:errorcluster, "Trap Pos FB Int-Norm Signal"=w2415:fxp<+/-,16,1>)
        n1581 = local read "Differential FB?"() -> (w2420:bool)
        n1582 = case shown="False" w2420 {
          tunnel: [w2425 w2432] -> w2422
          tunnel: w2415 -> [w2423 w2432]
          frame False {
            n1583 = local read "Trap Pos FB Monitor\nT1 or T2"() -> (w2428:bool)
            n1584 = local read "Trap X AI1 (DMA)"() -> (w2431:T13)
            n1585 = Unbundle By Name(w2431) -> ("Set 1"=w2430:fxp<+/-,16,1>, "Set 2"=w2429:fxp<+/-,16,1>)
            n1586 = Select(t=w2430, s=w2428, f=w2429) -> (s? t:f=w2427:fxp<+/-,16,1>)
            n1587 = Not(x="Set SP Using...") -> (.not. x?=w2424:bool)
            n1588 = Select(t=w2423, s=w2424, f=w2427) -> (s? t:f=w2425:fxp<+/-,16,1>)
          }
          frame True {
          }
        }
        n1589 = xnode "Read/Write Control"("FPGA VI Reference In"=w2417, "error in"=w2416, "Trap Pos. FB SP"=w2422) -> ()  [unwired: 2 out]
        n1590 = local write "Trap Pos FB SP"(w2422) -> ()
      }
      event "Trap Pos. FB Out Scale 2^n": Value Change {
        n1591 = event-data() -> ()  [unwired: 7 out]
        n1592 = Scale By Power Of 2(n="Trap Pos. FB Out Scale 2^n", x=ext 1.0) -> (x*2^n=w2433:ext)
        n1593 = property on="Trap Pos. FB Mult Factor" class="DigNum (strict)"("Val(Sgnl)"=w2433) -> ()  [unwired: 2 in, 2 out]
      }
      event "Trap Pos FB Int Count": Value Change {
        n1594 = event-data() -> ()  [unwired: 7 out]
        n1595 = xnode "Read/Write Control"("FPGA VI Reference In"=w2438, "error in"=w2437, "Trap Pos FB Int Count"="Trap Pos FB Int Count") -> ()  [unwired: 2 out]
      }
    }
    "error out 2" <- w1351
    n1596 = node-c288() -> ()  [unwired: 2 out]
  }
  n1597 = timed-loop "Mouse control: trap position (AOM deflection), set confocal spot from image" {
    tunnel: [w2440] -> w182
    tunnel: w50 -> [w2439]
    timing: w94 -> [_]
    timing-out: [_] -> w93
    stop <- w2440 stop-if-true
    n1598 = node-c288() -> ()  [unwired: 2 out]
    n1599 = event shown="[0] \"Pane\": Mouse Down" {
      selector: _ -> [_ _]
      dyn-events: _ -> [_ _]
      timeout: _ -> [_ _]
      tunnel: w2439 -> [w2443 _]
      event Mouse Down {
        n1600 = event-data() -> ("Time"=w2445:u32, "Coords"=w2444:T7, "Button"=w2446:u16)  [unwired: 6 out]
        n1601 = case shown="1" w2446 {
          tunnel: w2445 -> [_ _ w2549]
          tunnel: w2444 -> [_ w2483 w2547]
          tunnel: w2443 -> [_ _ w2545]
          frame 0, Default {
          }
          frame 1 {
            n1602 = property on="APD 2" class="ImageControl"() -> ("Displayed Image Position"=w2453:cluster{"Left":i32, "Top":i32})  [unwired: 2 in, 2 out]
            n1603 = property on="APD 1" class="ImageControl"() -> ("Displayed Image Position"=w2482:cluster{"Left":i32, "Top":i32})  [unwired: 2 in, 2 out]
            n1604 = property on="Detection Laser X" class="ImageControl"() -> ("Displayed Image Position"=w2479:cluster{"Left":i32, "Top":i32})  [unwired: 2 in, 2 out]
            n1605 = property on="Detection Laser Y" class="ImageControl"() -> ("Displayed Image Position"=w2478:cluster{"Left":i32, "Top":i32})  [unwired: 2 in, 2 out]
            n1606 = property on="APD 2" class="ImageControl"() -> ("Displayed Image Size"=w2452:cluster{"Width":u32, "Height":u32})  [unwired: 2 in, 2 out]
            n1607 = property on="APD 1" class="ImageControl"() -> ("Displayed Image Size"=w2480:cluster{"Width":u32, "Height":u32})  [unwired: 2 in, 2 out]
            n1608 = property on="Detection Laser X" class="ImageControl"() -> ("Displayed Image Size"=w2481:cluster{"Width":u32, "Height":u32})  [unwired: 2 in, 2 out]
            n1609 = property on="Detection Laser Y" class="ImageControl"() -> ("Displayed Image Size"=w2477:cluster{"Width":u32, "Height":u32})  [unwired: 2 in, 2 out]
            n1610 = Unbundle By Name(w2452) -> ("Width"=w2449:u32, "Height"=w2448:u32)
            n1611 = Unbundle By Name(w2453) -> ("Left"=w2451:i32, "Top"=w2450:i32)
            n1612 = Unbundle By Name(w2480) -> ("Width"=w2474:u32, "Height"=w2473:u32)
            n1613 = Unbundle By Name(w2481) -> ("Width"=w2470:u32, "Height"=w2469:u32)
            n1614 = Unbundle By Name(w2477) -> ("Width"=w2466:u32, "Height"=w2465:u32)
            n1615 = Unbundle By Name(w2482) -> ("Left"=w2476:i32, "Top"=w2475:i32)
            n1616 = Unbundle By Name(w2479) -> ("Left"=w2472:i32, "Top"=w2471:i32)
            n1617 = Unbundle By Name(w2478) -> ("Left"=w2468:i32, "Top"=w2467:i32)
            n1618 = Bundle("Left"=w2451, "Top"=w2450, "Width"=w2449, "Height"=w2448) -> (w2447:T29)  [unwired: 1 in]
            n1619 = Bundle("Left"=w2476, "Top"=w2475, "Width"=w2474, "Height"=w2473) -> (w2464:T29)  [unwired: 1 in]
            n1620 = Bundle("Left"=w2472, "Top"=w2471, "Width"=w2470, "Height"=w2469) -> (w2463:T29)  [unwired: 1 in]
            n1621 = Bundle("Left"=w2468, "Top"=w2467, "Width"=w2466, "Height"=w2465) -> (w2462:T29)  [unwired: 1 in]
            n1622 = Build Cluster Array(w2447, w2464, w2463, w2462) -> (w2461:T30)
            n1623 = for {
              tunnel: w2483 -> [w2494]
              tunnel: w2461 -> [w2495] mode=indexing
              shift-right: [w2492] -> w2459
              shift-left: TRUE -> [w2493]
              shift-right: [w2491] -> w2457
              shift-left: _ -> [w2487]
              shift-right: [w2490] -> w2456
              shift-left: _ -> [w2486]
              shift-right: [w2489] -> w2455
              shift-left: _ -> [w2485]
              shift-right: [w2488] -> w2454
              shift-left: _ -> [w2484]
              n1624 = case shown="True" w2493 {
                selector: w2493 -> [w2500 _]
                tunnel: w2495 -> [_ w2509]
                tunnel: w2494 -> [_ w2507]
                tunnel: [w2500 w2505] -> w2492
                tunnel: [w2499 w2504] -> w2491
                tunnel: [w2498 w2503] -> w2490
                tunnel: [w2497 w2502] -> w2489
                tunnel: [w2496 w2501] -> w2488
                tunnel: w2487 -> [w2499 _]
                tunnel: w2486 -> [w2498 _]
                tunnel: w2485 -> [w2497 _]
                tunnel: w2484 -> [w2496 _]
                frame False {
                }
                frame True {
                  n1625 = Unbundle(w2509) -> (w2508:T29)
                  n1626 = call "isclickinwindow.vi"("Image Param"=w2508, "Point32"=w2507) -> ("4 Y"=w2501:i32, "3 Height"=w2502:i32, "2 X"=w2503:i32, "1 Width"=w2504:i32, "In image?"=w2506:bool)  [unwired: 1 in]
                  n1627 = Not(x=w2506) -> (.not. x?=w2505:bool)
                }
              }
            }
            n1628 = Not(x=w2459) -> (.not. x?=w2458:bool)
            n1629 = case shown="True" w2458 {
              tunnel: w2456 -> [_ w2522]
              tunnel: w2454 -> [_ w2521]
              tunnel: w2457 -> [_ w2520]
              tunnel: w2455 -> [_ w2519]
              frame False {
              }
              frame True {
                w2515 = FALSE ("Get Point")
                n1630 = local read "Scan lines (y)"() -> (w2524:u64)
                n1631 = local read "Actual MCL Inc (V)"() -> (w2516:dbl)
                n1632 = local read "Scan steps (MCL)"() -> (w2523:u64)
                n1633 = Divide "Y Pix/step"(x=w2519, y=w2524) -> (x/y=w2531:dbl)
                n1634 = Divide "Y V/pix"(x=w2516, y=w2531) -> (x/y=w2530:dbl)
                n1635 = Divide "Y half step offset"(x=w2516, y=2.0) -> (x/y=w2532:dbl)
                n1636 = Divide "X pix/step"(x=w2520, y=w2523) -> (x/y=w2529:dbl)
                n1637 = Negate(x=w2532) -> (-x=w2533:dbl)
                n1638 = local read "Initial Y"() -> (w2539:dbl)
                n1639 = Multiply(x=w2521, y=w2530) -> (x*y=w2540:dbl)
                n1640 = Divide "X half step offset"(x=w2516, y=2.0) -> (x/y=w2526:dbl)
                n1641 = Divide "X V/pix"(x=w2516, y=w2529) -> (x/y=w2528:dbl)
                n1642 = Multiply(x=w2516, y=w2523) -> (x*y=w2535:dbl)
                n1643 = Compound Arithmetic op=ADD(w2533, w2540, w2539) -> (w2517:dbl)
                "Pointer Y (V)" <- w2517
                n1644 = Multiply(x=w2528, y=w2522) -> (x*y=w2537:dbl)
                n1645 = Negate(x=w2526) -> (-x=w2525:dbl)
                n1646 = local read "Initial X"() -> (w2538:dbl)
                n1647 = Negate(x=w2537) -> (-x=w2536:dbl)
                n1648 = Compound Arithmetic op=ADD(w2525, w2535, w2538, w2536) -> (w2518:dbl)
                "Pointer X (V)" <- w2518
                n1649 = Or(x="Set X Only", y="Set Confocal Spot (X-Y)") -> (x .or. y?=w2511:bool)
                n1650 = Or(x="Set Confocal Spot (X-Y)", y="Set Y Only") -> (x .or. y?=w2510:bool)
                n1651 = case shown="True" w2511 {
                  tunnel: w2518 -> [_ w2541]
                  frame False {
                  }
                  frame True {
                    n1652 = property on="AO2" class="Slide (strict)"("Val(Sgnl)"=w2541) -> ()  [unwired: 2 in, 2 out]
                  }
                }
                n1653 = case shown="True" w2510 {
                  tunnel: w2517 -> [_ w2542]
                  frame False {
                  }
                  frame True {
                    n1654 = property on="AO1" class="Slide (strict)"("Val(Sgnl)"=w2542) -> ()  [unwired: 2 in, 2 out]
                  }
                }
                n1655 = local write "Set Confocal Spot (X-Y)"(w2515) -> ()
                n1656 = local write "Set X Only"(w2515) -> ()
                n1657 = local write "Set Y Only"(w2515) -> ()
              }
            }
          }
          frame 3 {
            n1658 = local read "BD 2 Frequency 1 (MHz)"() -> (w2543:dbl)
            n1659 = local read "BD 1 Frequency 1 (MHz)"() -> (w2544:dbl)
            n1660 = local write "Manipulating Trap"(TRUE ("Manipulating Trap")) -> ()
            n1661 = local write "Coords"(T7 {"Horizontal"=0, "Vertical"=0} ("Coords")) -> ()
            n1662 = while {
              tunnel: w2549 -> [w2554]
              tunnel: w2547 -> [w2553]
              tunnel: w2545 -> [w2552]
              tunnel: w2544 -> [w2551]
              tunnel: w2543 -> [w2550]
              stop <- w2555 stop-if-true
              n1663 = event shown="[0] \"Pane\": Mouse Move" {
                selector: _ -> [_ _]
                dyn-events: _ -> [_ _]
                timeout: _ -> [_ _]
                tunnel: ["Force Manip Abort" w2619] -> w2555
                tunnel: w2554 -> [w2562 _]
                tunnel: w2553 -> [w2560 _]
                tunnel: w2552 -> [w2559 _]
                tunnel: w2551 -> [w2558 _]
                tunnel: w2550 -> [w2557 _]
                event Mouse Move {
                  n1664 = event-data() -> ("Time"=w2563:u32, "Coords"=w2564:T7)  [unwired: 3 out]
                  n1665 = Less?(x=w2563, y=w2562) -> (x < y?=w2561:bool)
                  n1666 = case "Makes sure old motion events prior to mouse click aren't used" shown="False" w2561 {
                    tunnel: w2564 -> [w2606 _]
                    tunnel: w2560 -> [w2607 _]
                    tunnel: w2559 -> [w2584 _]
                    tunnel: w2558 -> [w2580 _]
                    tunnel: w2557 -> [w2579 _]
                    frame False {
                      n1667 = Subtract(x=w2606, y=w2607) -> (x-y=w2605:T7)
                      "Coords" <- w2605
                      n1668 = local read "Y RF Frequency Limits (MHz)"() -> (w2565:T16)
                      n1669 = To Double Precision Float(number=w2605) -> (double precision float=w2604:cluster{"Horizontal":dbl, "Vertical":dbl})
                      n1670 = Multiply(x=cluster{"Horizontal":dbl, "Vertical":dbl} {"Horizontal"=-1.0, "Vertical"=1.0}, y="Manipulation Scaling") -> (x*y=w2600:cluster{"Horizontal":dbl, "Vertical":dbl})
                      n1671 = local read "X RF Frequency Limits (MHz)"() -> (w2566:T16)
                      n1672 = Multiply(x=w2604, y=w2600) -> (x*y=w2602:cluster{"Horizontal":dbl, "Vertical":dbl})
                      n1673 = Unbundle By Name(w2602) -> ("Horizontal"=w2597:dbl, "Vertical"=w2601:dbl)
                      n1674 = Unbundle By Name(w2565) -> ("Maximum"=w2568:dbl, "Minimum"=w2567:dbl)
                      n1675 = Boolean To (0,1)(Boolean="Manip. X?") -> (0, 1=w2595:i16)
                      n1676 = Boolean To (0,1)(Boolean="Manip. Y?") -> (0, 1=w2592:i16)
                      n1677 = local read "BD 1 Frequency 2 (MHz)"() -> (w2582:dbl)
                      n1678 = Multiply(x=w2601, y=w2592) -> (x*y=w2594:dbl)
                      n1679 = Multiply(x=w2595, y=w2597) -> (x*y=w2598:dbl)
                      n1680 = local read "BD 2 Frequency 2 (MHz)"() -> (w2581:dbl)
                      n1681 = Unbundle By Name(w2566) -> ("Maximum"=w2570:dbl, "Minimum"=w2569:dbl)
                      n1682 = Add(x=w2579, y=w2594) -> (x+y=w2572:dbl)
                      n1683 = Add(x=w2580, y=w2598) -> (x+y=w2574:dbl)
                      n1684 = In Range and Coerce(upper limit=w2570, x=w2574, lower limit=w2569) -> (coerced(x)=w2573:dbl)  [unwired: 1 out]
                      n1685 = In Range and Coerce(upper limit=w2568, x=w2572, lower limit=w2567) -> (coerced(x)=w2571:dbl)  [unwired: 1 out]
                      n1686 = Subtract(x=w2573, y=w2582) -> (x-y=w2591:dbl)
                      n1687 = Subtract(x=w2571, y=w2581) -> (x-y=w2590:dbl)
                      n1688 = Square(x=w2591) -> (x^2=w2589:dbl)
                      n1689 = Square(x=w2590) -> (x^2=w2588:dbl)
                      n1690 = Add(x=w2589, y=w2588) -> (x+y=w2587:dbl)
                      n1691 = Square Root(x=w2587) -> (sqrt(x)=w2583:dbl)
                      n1692 = In Range and Coerce(upper limit="Limit Max (MHz)", x=w2583, lower limit="Limit Min (MHz)") -> (In Range?=w2576:bool)  [unwired: 1 out]
                      n1693 = Not(x="Limits Enable") -> (.not. x?=w2575:bool)
                      n1694 = Or(x=w2576, y=w2575) -> (x .or. y?=w2577:bool)
                      n1695 = case shown="True" w2577 {
                        tunnel: w2584 -> [_ w2617]
                        tunnel: w2583 -> [_ w2608]
                        tunnel: w2573 -> [_ w2615]
                        tunnel: w2582 -> [_ w2614]
                        tunnel: w2571 -> [_ w2613]
                        tunnel: w2581 -> [_ w2612]
                        tunnel: w2566 -> [_ w2610]
                        tunnel: w2565 -> [_ w2609]
                        frame False {
                        }
                        frame True {
                          n1696 = local read "BD 1 Frequency 3 (MHz)"() -> (w2616:dbl)
                          n1697 = local read "BD 2 Frequency 3 (MHz)"() -> (w2611:dbl)
                          n1698 = local write "Trap Delta (MHz)"(w2608) -> ()
                          n1699 = call "set RF board frequency - interlace.vi"("Board 2 Frequency Limits"=w2609, "Board 1 Frequency Limits"=w2610, "FPGA VI Reference In"=w2617, "Board 2 Frequency 3 (MHz)"=w2611, "Board 1 Frequency 3 (MHz)"=w2616, "Board 2 Frequency 2 (MHz)"=w2612, "Board 2 Frequency 1 (MHz)"=w2613, "Board 1 Frequency 2 (MHz)"=w2614, "Board 1 Frequency 1  (MHz)"=w2615) -> ()  [unwired: 1 in, 2 out]
                          n1700 = local write "BD 2 Frequency 1 (MHz)"(w2613) -> ()
                          n1701 = local write "BD 1 Frequency 1 (MHz)"(w2615) -> ()
                        }
                      }
                    }
                    frame True {
                    }
                  }
                }
                event Mouse Up {
                  n1702 = event-data() -> ("Button"=w2618:u16)  [unwired: 8 out]
                  n1703 = case shown="3" w2618 {
                    tunnel: [FALSE TRUE] -> w2619
                    frame 0, Default {
                    }
                    frame 3 {
                      n1704 = local read "Trap Delta (MHz)"() -> (w2621:dbl)
                      n1705 = property on="Initial delta (MHz)" class="DigNum (strict)"("Val(Sgnl)"=w2621) -> ()  [unwired: 2 in, 2 out]
                      n1706 = local write "Manipulating Trap"(FALSE ("Manipulating Trap")) -> ()
                    }
                  }
                }
              }
            }
          }
        }
      }
      event Mouse Move {
        n1707 = event-data() -> ()  [unwired: 6 out]
      }
    }
    n1708 = local read "Stop All"() -> (w2440:bool)
    n1709 = node-c288() -> ()  [unwired: 2 out]
  }
  n1710 = flat-sequence "Video" {
    tunnel: [w2632] -> w80
    tunnel: w80 -> [w2673]
    frame #0 {
      n1711 = while {
        stop <- w2625 continue-if-true
        n1712 = call "Close Video Capture.vi"() -> ("error code OUT"=w2627:i32)
        n1713 = Equal?(x=w2627, y=0) -> (x = y?=w2625:bool)
      }
      n1714 = local write "Stop All"(FALSE ("Stop All")) -> ()
    }
    frame #1 {
      n1715 = call "DMR_Init.vi"() -> ()  [unwired: 3 out]
    }
    frame #2 {
      # "Setting the destination format to Mono8 makes sure that the image can be displayed in the intensity plot."
      n1716 = call "DMR_GetDevice.vi"("search string IN"="DE019116701") -> ("device handle OUT"=w2650:i32)  [unwired: 4 in, 2 out]
      n1717 = call "DMR_OpenDevice.vi"("device handle IN"=w2650) -> ("driver handle OUT"=w2633:i32)  [unwired: 4 out]
      n1718 = call "DMR_FindList.vi"("flags IN"=u32 0 ("flags"), "list name IN"="" ("String"), "list type IN"=T31."camera descriptions", "driver handle IN"=w2633) -> ("list handle OUT"=w2636:i32)  [unwired: 2 out]
      n1719 = call "DMR_FindList.vi"("flags IN"=u32 0 ("flags"), "list name IN"="Base", "list type IN"=T31."setting", "driver handle IN"=w2633) -> ("list handle OUT"=w2634:i32)  [unwired: 2 out]
      n1720 = call "OBJ_GetHandle.vi"("object name IN"="VideoStandard", "list handle IN"=w2636) -> ("object handle OUT"=w2630:i32)  [unwired: 3 out]
      n1721 = call "OBJ_GetHandle.vi"("object name IN"="PixelFormat", "list handle IN"=w2634) -> ("object handle OUT"=w2644:i32)  [unwired: 3 out]
      n1722 = call "OBJ_SetS.vi"("value index IN"=0, "value IN"="NTSC M", "object handle IN"=w2630) -> ()  [unwired: 2 out]
      n1723 = call "OBJ_SetS.vi"("value index IN"=0, "value IN"="Mono8" ("value"), "object handle IN"=w2644) -> ()  [unwired: 2 out]
      n1724 = call "OBJ_GetHandle.vi"("object name IN"="VideoChannel", "list handle IN"=w2634) -> ("object handle OUT"=w2640:i32)  [unwired: 3 out]
      n1725 = while {
        tunnel: [w2655] -> w2632
        tunnel: w2633 -> [w2652]
        stop <- w2653 continue-if-true
        n1726 = call "DMR_ImageRequestSingle.vi"("request control IN"=0, "driver handle IN"=w2652) -> ("error code OUT"=w2654:i32, "driver handle OUT"=w2655:i32)  [unwired: 2 out]
        n1727 = Equal To 0?(x=w2654) -> (x = 0?=w2653:bool)
      }
      n1728 = call "OBJ_SetI.vi"("value index IN"=0, "value IN"=3 ("Video channel"), "object handle IN"=w2640) -> ()  [unwired: 2 out]
    }
    frame #3 {
      w2661 = T17 0 items=["Grayscale (U8)", "Grayscale (I16)", "Grayscale (SGL)", "Complex (CSG)", "RGB (U32)", "HSL (U32)", "RGB (U64)"] ("Image Type")
